vi "Connect error.vi"(9 "LastError":string, 10 "PCAN Read error":string, 11 "source":string) -> (1 "LastError out":string)   [LabVIEW 2020]
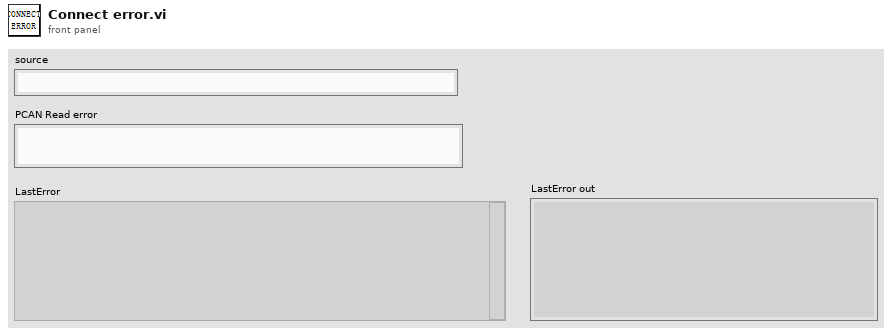
[diagram p1: front panel]
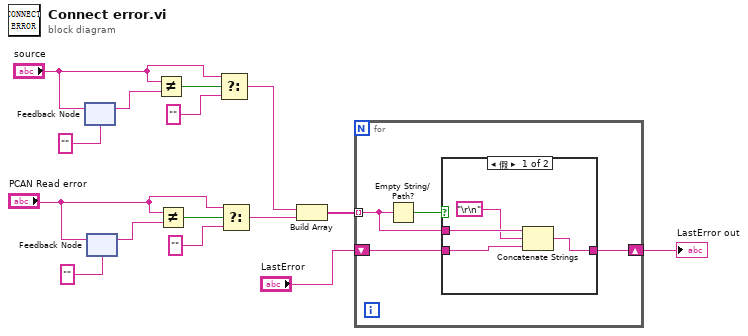
[diagram p0: block diagram]
diagram:
  n1 = feedback-in #1("source") -> ()
  n2 = feedback #1("" ("source")) -> (w14:string)
  n3 = feedback #2("" ("source")) -> (w8:string)
  n4 = feedback-in #2("PCAN Read error") -> ()
  n5 = Not Equal?(x="source", y=w14) -> (x != y?=w13:bool)
  n6 = Not Equal?(x="PCAN Read error", y=w8) -> (x != y?=w9:bool)
  n7 = Select(t="source", s=w13, f="") -> (s? t:f=w4:string)
  n8 = Select(t="PCAN Read error", s=w9, f="") -> (s? t:f=w5:string)
  n9 = Build Array(w4, w5) -> (w3:string[])
  n10 = for {
    tunnel: w3 -> [w17] mode=indexing
    shift-right: [w16] -> w1
    shift-left: "LastError" -> [w18]
    n11 = Empty String/Path?(string/path=w17) -> (empty?=w19:bool)
    n12 = case shown="假" w19 {
      tunnel: w18 -> [w22 w24]
      tunnel: w17 -> [w23 _]
      tunnel: [w20 w24] -> w16
      frame False {
        n13 = Concatenate Strings(w23, "\r\n", w22) -> (w20:string)
      }
      frame True {
      }
    }
  }
  "LastError out" <- w1
